vi "pmu_Check Input Data Error.vi"(0 "data in":T3, 1 "frequency configuration":T2={"channel index"=0, "nominal Fs/actual Fs"=1.0}, 2 "reset? (F)":bool, 5 "elements need to read":u32, 7 "max time error [s]":dbl=1e-07 format="%#_15f", 9 "system info in":refnum<class "PMU System Info.lvclass">, 11 "error in (no error)":errorcluster, 12 "GPS information":T1[](array[typedef])) -> (10 "system info out":refnum<class "PMU System Info.lvclass">, 15 "error out":errorcluster)   [LabVIEW 2012, in "NI_EP_PMU.lvlib"]
uses:
  <vilib>/addons/Electrical Power/PMU/NI_EP_PMU.lvlib
  <vilib>/addons/Electrical Power/PMU/Common/Controls/pmu_Phasor Measurement Data.ctl
  <vilib>/addons/Electrical Power/PMU/Common/Controls/pmu_GPS Info.ctl
  <vilib>/addons/Electrical Power/PMU/Common/Classes/PMU System Info/PMU System Info.lvclass
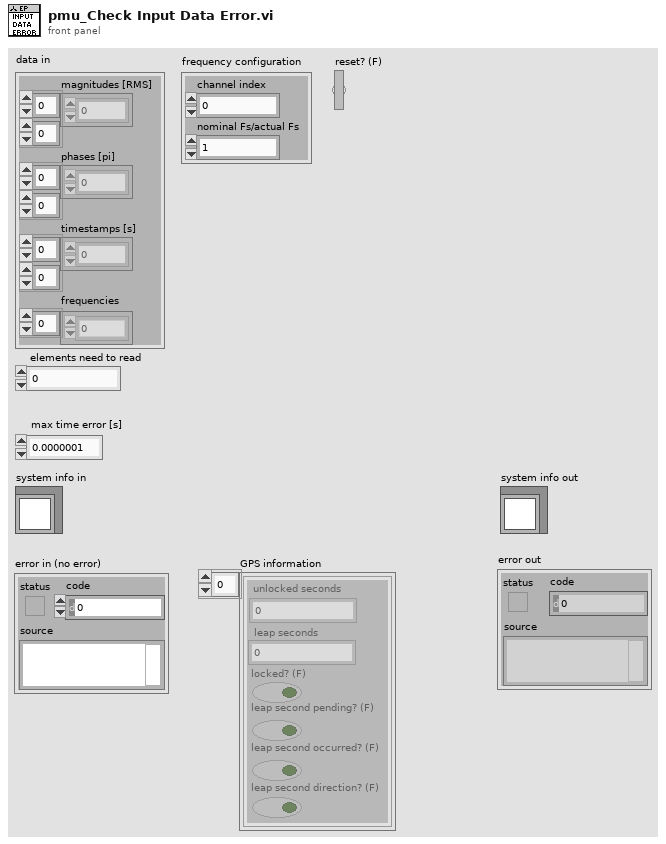
[diagram p1: front panel]
types:
  T1 = typedef "NI_EP_PMU.lvlib/pmu_GPS Info.ctl" = cluster{"unlocked seconds":u32, "leap seconds":i8, "locked? (F)":bool, "leap second pending? (F)":bool, "leap second occurred? (F)":bool, "leap second direction? (F)":bool}
  T2 = cluster{"channel index":i32, "nominal Fs/actual Fs":dbl}
  T3 = typedef "NI_EP_PMU.lvlib/pmu_Phasor Measurement Data.ctl" = cluster{"magnitudes [RMS]":dbl[][], "phases [pi]":dbl[][], "timestamps [s]":dbl[][], "frequencies":dbl[]}
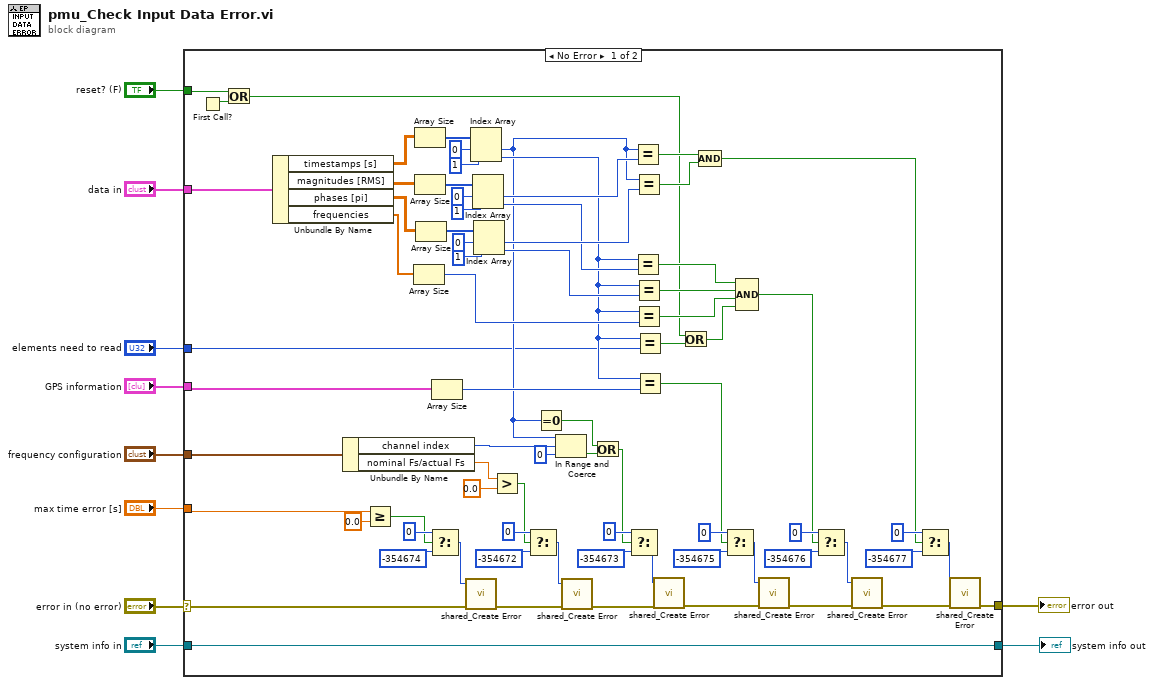
[diagram p0: block diagram]
diagram:
  n1 = case shown="No Error" "error in (no error)" {
    selector: "error in (no error)" -> [w15 w86]
    tunnel: "data in" -> [w81 _]
    tunnel: "elements need to read" -> [w16 _]
    tunnel: "reset? (F)" -> [w59 _]
    tunnel: "max time error [s]" -> [w58 _]
    tunnel: "GPS information" -> [w56 _]
    tunnel: "frequency configuration" -> [w53 _]
    tunnel: "system info in" -> [w14 w87]
    tunnel: [w14 w87] -> w3
    tunnel: [w19 w86] -> w1
    frame No Error {
      n2 = First Call?() -> (First Call?: T/F=w60:bool)
      n3 = Or(x=w59, y=w60) -> (x .or. y?=w11:bool)
      n4 = Unbundle By Name(w81) -> ("timestamps [s]"=w84:dbl[][], "magnitudes [RMS]"=w83:dbl[][], "phases [pi]"=w82:dbl[][], "frequencies"=w85:dbl[])
      n5 = Unbundle By Name(w53) -> ("channel index"=w52:i32, "nominal Fs/actual Fs"=w49:dbl)
      n6 = Greater Or Equal?(x=w58, y=0.0) -> (x >= y?=w18:bool)
      n7 = Array Size(array=w85) -> (size(s)=w61:i32)
      n8 = Array Size(array=w84) -> (size(s)=w80:i32[])
      n9 = Array Size(array=w83) -> (size(s)=w75:i32[])
      n10 = Array Size(array=w82) -> (size(s)=w72:i32[])
      n11 = Select(t=0 ("lower limit"), s=w18, f=-354674) -> (s? t:f=w44:i32)
      n12 = Array Size(array=w56) -> (size(s)=w55:i32)
      n13 = call <vilib>:"shared_Create Error.vi"("error in (no error)"=w15, "error code (0)"=w44) -> ("error out"=w41:errorcluster)  [unwired: 9 in]
      n14 = Index Array(array=w80, index #1=0 ("index"), index #2=1 ("index")) -> (element #1=w48:i32, element #2=w54:i32)
      n15 = Index Array(array=w75, index #1=0 ("index"), index #2=1 ("index")) -> (element #1=w71:i32, element #2=w67:i32)
      n16 = Index Array(array=w72, index #1=0 ("index"), index #2=1 ("index")) -> (element #1=w70:i32, element #2=w66:i32)
      n17 = Greater?(x=w49, y=0.0) -> (0:w17:bool)
      n18 = Select(t=0 ("lower limit"), s=w17, f=-354672) -> (s? t:f=w43:i32)
      n19 = Equal To 0?(x=w48) -> (x = 0?=w46:bool)
      n20 = In Range and Coerce(upper limit=w48, x=w52, lower limit=0) -> (In Range?=w47:bool)  [unwired: 1 out]
      n21 = call <vilib>:"shared_Create Error.vi"("error in (no error)"=w41, "error code (0)"=w43) -> ("error out"=w35:errorcluster)  [unwired: 9 in]
      n22 = Or(x=w46, y=w47) -> (x .or. y?=w34:bool)
      n23 = Select(t=0 ("lower limit"), s=w34, f=-354673) -> (s? t:f=w36:i32)
      n24 = Equal?(x=w48, y=w71) -> (x = y?=w69:bool)
      n25 = Equal?(x=w54, y=w67) -> (x = y?=w62:bool)
      n26 = Equal?(x=w48, y=w70) -> (x = y?=w68:bool)
      n27 = Equal?(x=w54, y=w66) -> (x = y?=w63:bool)
      n28 = Equal?(x=w54, y=w61) -> (x = y?=w64:bool)
      n29 = Equal?(x=w54, y=w16) -> (x = y?=w65:bool)
      n30 = Equal?(x=w54, y=w55) -> (x = y?=w29:bool)
      n31 = call <vilib>:"shared_Create Error.vi"("error in (no error)"=w35, "error code (0)"=w36) -> ("error out"=w33:errorcluster)  [unwired: 9 in]
      n32 = Or(x=w11, y=w65) -> (x .or. y?=w12:bool)
      n33 = Compound Arithmetic op=AND(w69, w68) -> (w20:bool)
      n34 = Select(t=0 ("lower limit"), s=w29, f=-354675) -> (s? t:f=w30:i32)
      n35 = Compound Arithmetic op=AND(w62, w63, w64, w12) -> (w13:bool)
      n36 = call <vilib>:"shared_Create Error.vi"("error in (no error)"=w33, "error code (0)"=w30) -> ("error out"=w28:errorcluster)  [unwired: 9 in]
      n37 = Select(t=0 ("lower limit"), s=w13, f=-354676) -> (s? t:f=w25:i32)
      n38 = call <vilib>:"shared_Create Error.vi"("error in (no error)"=w28, "error code (0)"=w25) -> ("error out"=w24:errorcluster)  [unwired: 9 in]
      n39 = Select(t=0 ("lower limit"), s=w20, f=-354677) -> (s? t:f=w21:i32)
      n40 = call <vilib>:"shared_Create Error.vi"("error in (no error)"=w24, "error code (0)"=w21) -> ("error out"=w19:errorcluster)  [unwired: 9 in]
    }
    frame Error {
    }
  }
  "error out" <- w1
  "system info out" <- w3
